vi "Keithley 2002 Reset.vi"(1 "reset/preset":bool, 2 "error in":T1, 3 "GPIB address":string="16") -> (0 "error out":T1)   [LabVIEW 2020]
doc: "This VI for the Keithley 2002 DMM allows the operator to send a \"reset\" or \"preset\" command to the unit. The differences between each of these is explained in full in the instruction manual."
panel:
  # "reset\npreset"
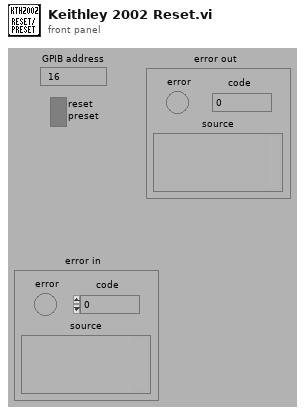
[diagram p1: front panel]
types:
  T1 = cluster{"error":bool, "code":i32, "source":string}
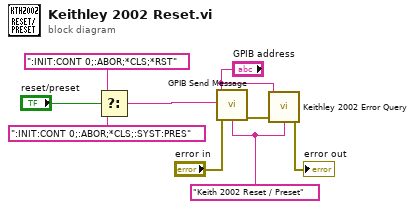
[diagram p0: block diagram]
diagram:
  w3 = "Keith 2002 Reset / Preset"
  n1 = Select(t=":INIT:CONT 0;:ABOR;*CLS;*RST", s="reset/preset", f=":INIT:CONT 0;:ABOR;*CLS;:SYST:PRES") -> (s? t:f=w8:string)
  n2 = call "GPIB Send Message.vi"("address string"="GPIB address", "write buffer"=w8, "source"=w3, "error in"="error in") -> ("error out"=w2:T1)  [unwired: 3 in, 2 out]
  n3 = call "Keithley 2002 Error Query.vi"("GPIB address"="GPIB address", "error in"=w2, "source"=w3) -> ("error out"=→"error out":T1)  [unwired: 2 out]
